vi "拉曼数据助手.vi"() -> ()   [LabVIEW 2020]
uses:
  <vilib>/Platform/TimedLoop/XDataNode/timing_clust.ctl
  <vilib>/Platform/TimedLoop/XDataNode/nitl_modes.ctl
  <vilib>/Platform/TimedLoop/XDataNode/wakeup.ctl
  <vilib>/picture/cartesn2.llb/XY Plot Type.ctl
  <vilib>/Instr/_visa.llb/VISA Configure Serial Port (Instr).vi
  <vilib>/Platform/TimedLoop/XDataNode/XDataNode.xnode
  <vilib>/Platform/TimedLoop/XDataNode/XDNodeRunTimeDep.lvlib
  <vilib>/Analysis/NI_AALPro.lvlib
  <vilib>/gmath/NI_Gmath.lvlib
panel:
  out "Window":bool
  out "配置文件路径":path
  out "偏移量":i32
  out "峰值范围":i32[][](array[numeric])
  out "λ picture":picture caption="新图片"
  out "pixel picture":picture
  in  "导出图像":bool
  in  "导出图像路路径":path caption="PNG图像文件路径"
  in  "自动寻峰":bool
  in  "关闭串口并退出":bool
  out "Debug状态":T1
  out "r^2":dbl caption="标定拟合 r" format="%.7g"
  in  "峰值波长":dbl[](array[numeric])=[0.0, 0.0]
  in  "峰值Pixel":dbl[](array[numeric])
  in  "自动转换":enum32{"Item 0", "Item 1"}(radio)
  out "波形XY图":T2
  in  "cartesian axis attributes":T3={"x minimum"=0.0, "x maximum"=0.0, "x log?"=FALSE, "x precision"=1, "x format"=enum."Decimal", "y minimum"=0.0, "y maximum"=0.0, "y log?"=FALSE, "y precision"=1, "y format"=enum."Decimal"} caption="直角坐标属性" {"x minimum" format="%0.2f"; "x maximum" format="%0.2f"; "y minimum" format="%0.2f"; "y maximum" format="%0.2f"}
  out "X轴":i32[](array[numeric])
  in  "导出文本":bool
  in  "数据存储路径":path=path "test.xlsx" caption="数据文件名"
  in  "暗背景扣除":bool
  in  "暗背景采集":bool
  out "暗背景":i64[](array[numeric])
  in  "确定":bool
  in  "时间单位":enum32{"Item 0", "Item 1"}(radio)
  in  "积分时间":dbl[unit]=0.1
  in  "Stop":bool
  out "采集状态":bool
  in  "波特率 (9600)":u32=9600 caption="波特率(9600)"
  in  "串口名":T4 caption="CCD检测器串口名"
  in  "开始":T5
  # "乙醇标定峰值 / pixel"
  # "2"
  # "-1"
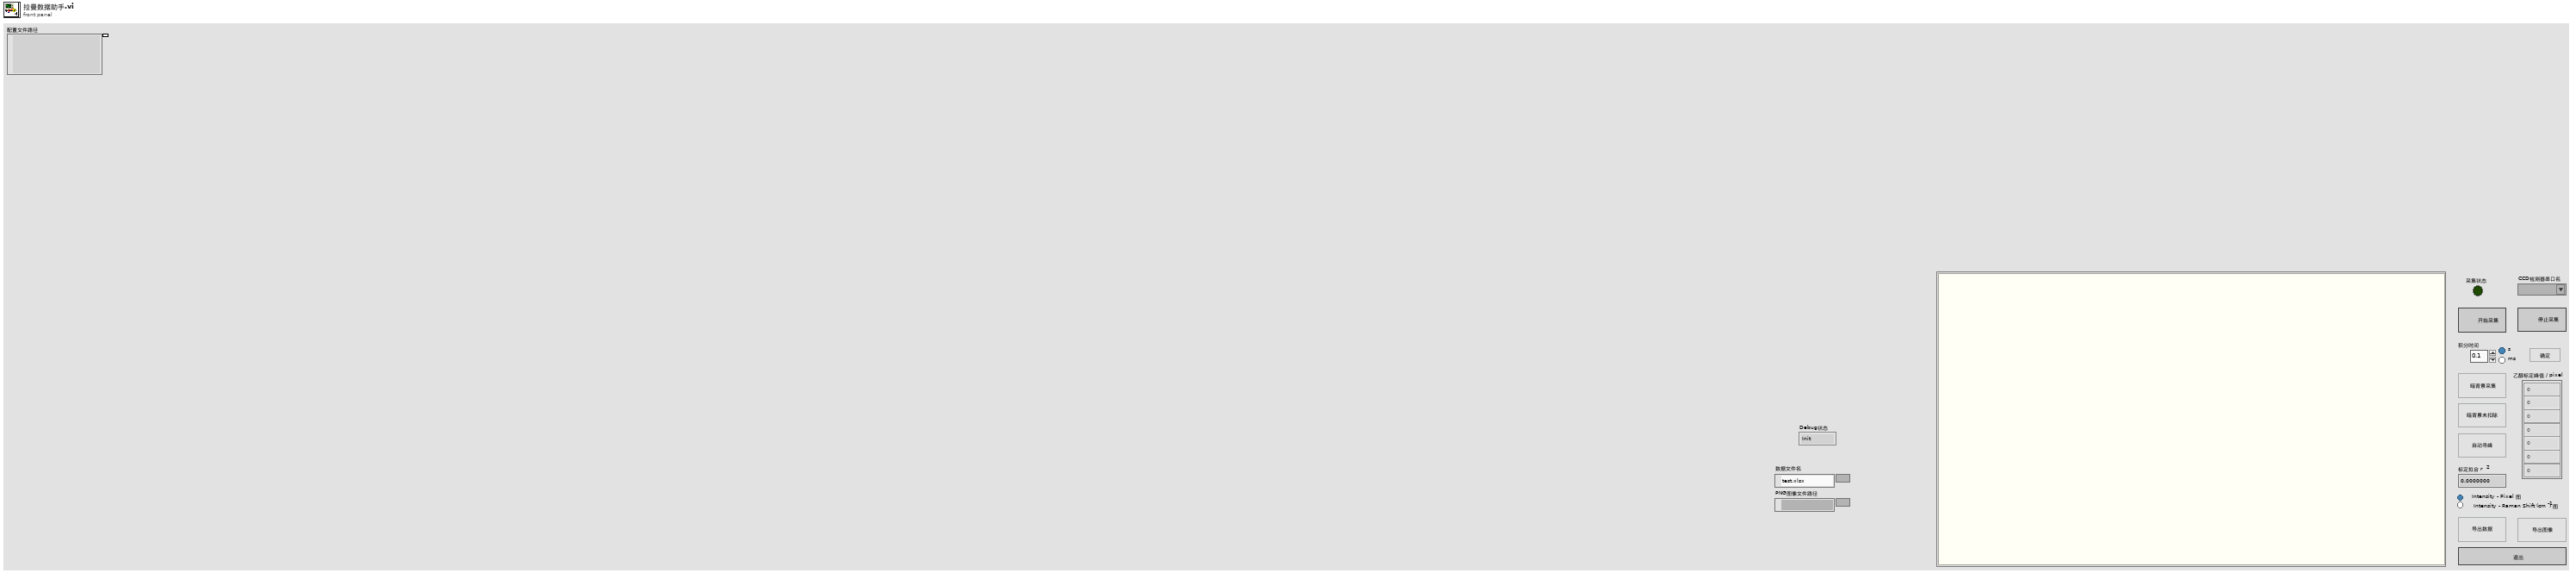
[diagram p1: front panel]
types:
  T1 = typedef "状态机.ctl" = enum16{"Init", "Wait", "GetData", "Exit"}
  T2 = typedef "？？.ctl" = picture
  T3 = cluster{"x minimum":dbl, "x maximum":dbl, "x log?":bool, "x precision":u8, "x format":enum8{"Decimal", "Scientific", "Engineering", "Binary", "Octal", "Hex"}, "y minimum":dbl, "y maximum":dbl, "y log?":bool, "y precision":u8, "y format":enum8{"Decimal", "Scientific", "Engineering", "Binary", "Octal", "Hex"}}
  T4 = typedef "控件 1.ctl" = refnum<visa-resource-name>
  T5 = typedef "1.ctl" = bool
  T6 = enum16{"open", "replace", "create", "open or create", "replace or create", "replace or create with confirmation"}
  T7 = cluster{"Font Name:":string, "Size":i16, "Strikeout?":bool, "Italic?":bool, "Underline?":bool, "Outline?":bool, "Shadow?":bool, "Bold?":bool}
  T8 = enum16{"User-specified Font", "Application Font", "System Font", "Dialog Font"}
  T9 = enum16{"None", "Stacked", "Clockwise", "Counterclockwise"}
  T10 = typedef "XY Plot Type.ctl" = enum16{"points", "squares", "circles", "connected points", "connected squares", "connected circles", "comb plot", "sized scatter plot", "sized-colored scatter plot", "min-max lines"}
  T11 = cluster{"plot color":u32, "XY plot type":T10, "baseline":dbl}
  T12 = cluster{"line color":u32, "text color":u32, "tick length(3)":i16, "crossing axes":bool, "visible grid?":bool}
  T13 = typedef "XDNodeRunTimeDep.lvlib/timing_clust.ctl" = cluster{"Expected End [f-1]":u64, "Actual End [f-1]":u64, "Finished Late? [f-1]":bool, "Expected End [i-1]":u64, "Actual End [i-1]":u64, "Finished Late? [i-1]":bool, "Expected Start [i]":u64, "Actual Start [i]":u64, "Expected Start [f]":u64, "Actual Start [f]":u64, "Source Name":string, "Structure Name":string, "Period":i64, "Deadline":i64, "Offset":i64, "Start":i64, "Priority":i32, "Timeout":i32, "Mode":T14, "Wakeup Reason":T15, "Error":errorcluster, "Source Type":string, "Secondary Source Type":string, "Global End Time":u64, "Global Start Time":u64, "Frame Duration":u64, "Iteration Duration":u64, "Assigned CPU":i32, "I/O Scan Engine Mode":u32}
  T14 = typedef "XDNodeRunTimeDep.lvlib/nitl_modes.ctl" = enum32{"No Change", "Process missed periods, maintain original phase", "Discard missed periods, maintain original phase", "Process missed periods, ignore original phase", "Discard missed periods, ignore original phase"}
  T15 = typedef "XDNodeRunTimeDep.lvlib/wakeup.ctl" = enum32{"Normal", "Aborted", "Asynchronous wakeup", "Timing source error", "Timed loop error", "Timeout"}
  T16 = cluster{i32, i32, i32, i32, i32, i32, i32, i32, i32, i32, i32, i32, i32, i32}
  T17 = typedef "imagedata.ctl" = cluster{"image type":i32, "image depth":i32, "image":u8[], "mask":u8[], "colors":u32[], "Rectangle":cluster{"left":i16, "top":i16, "right":i16, "bottom":i16}}
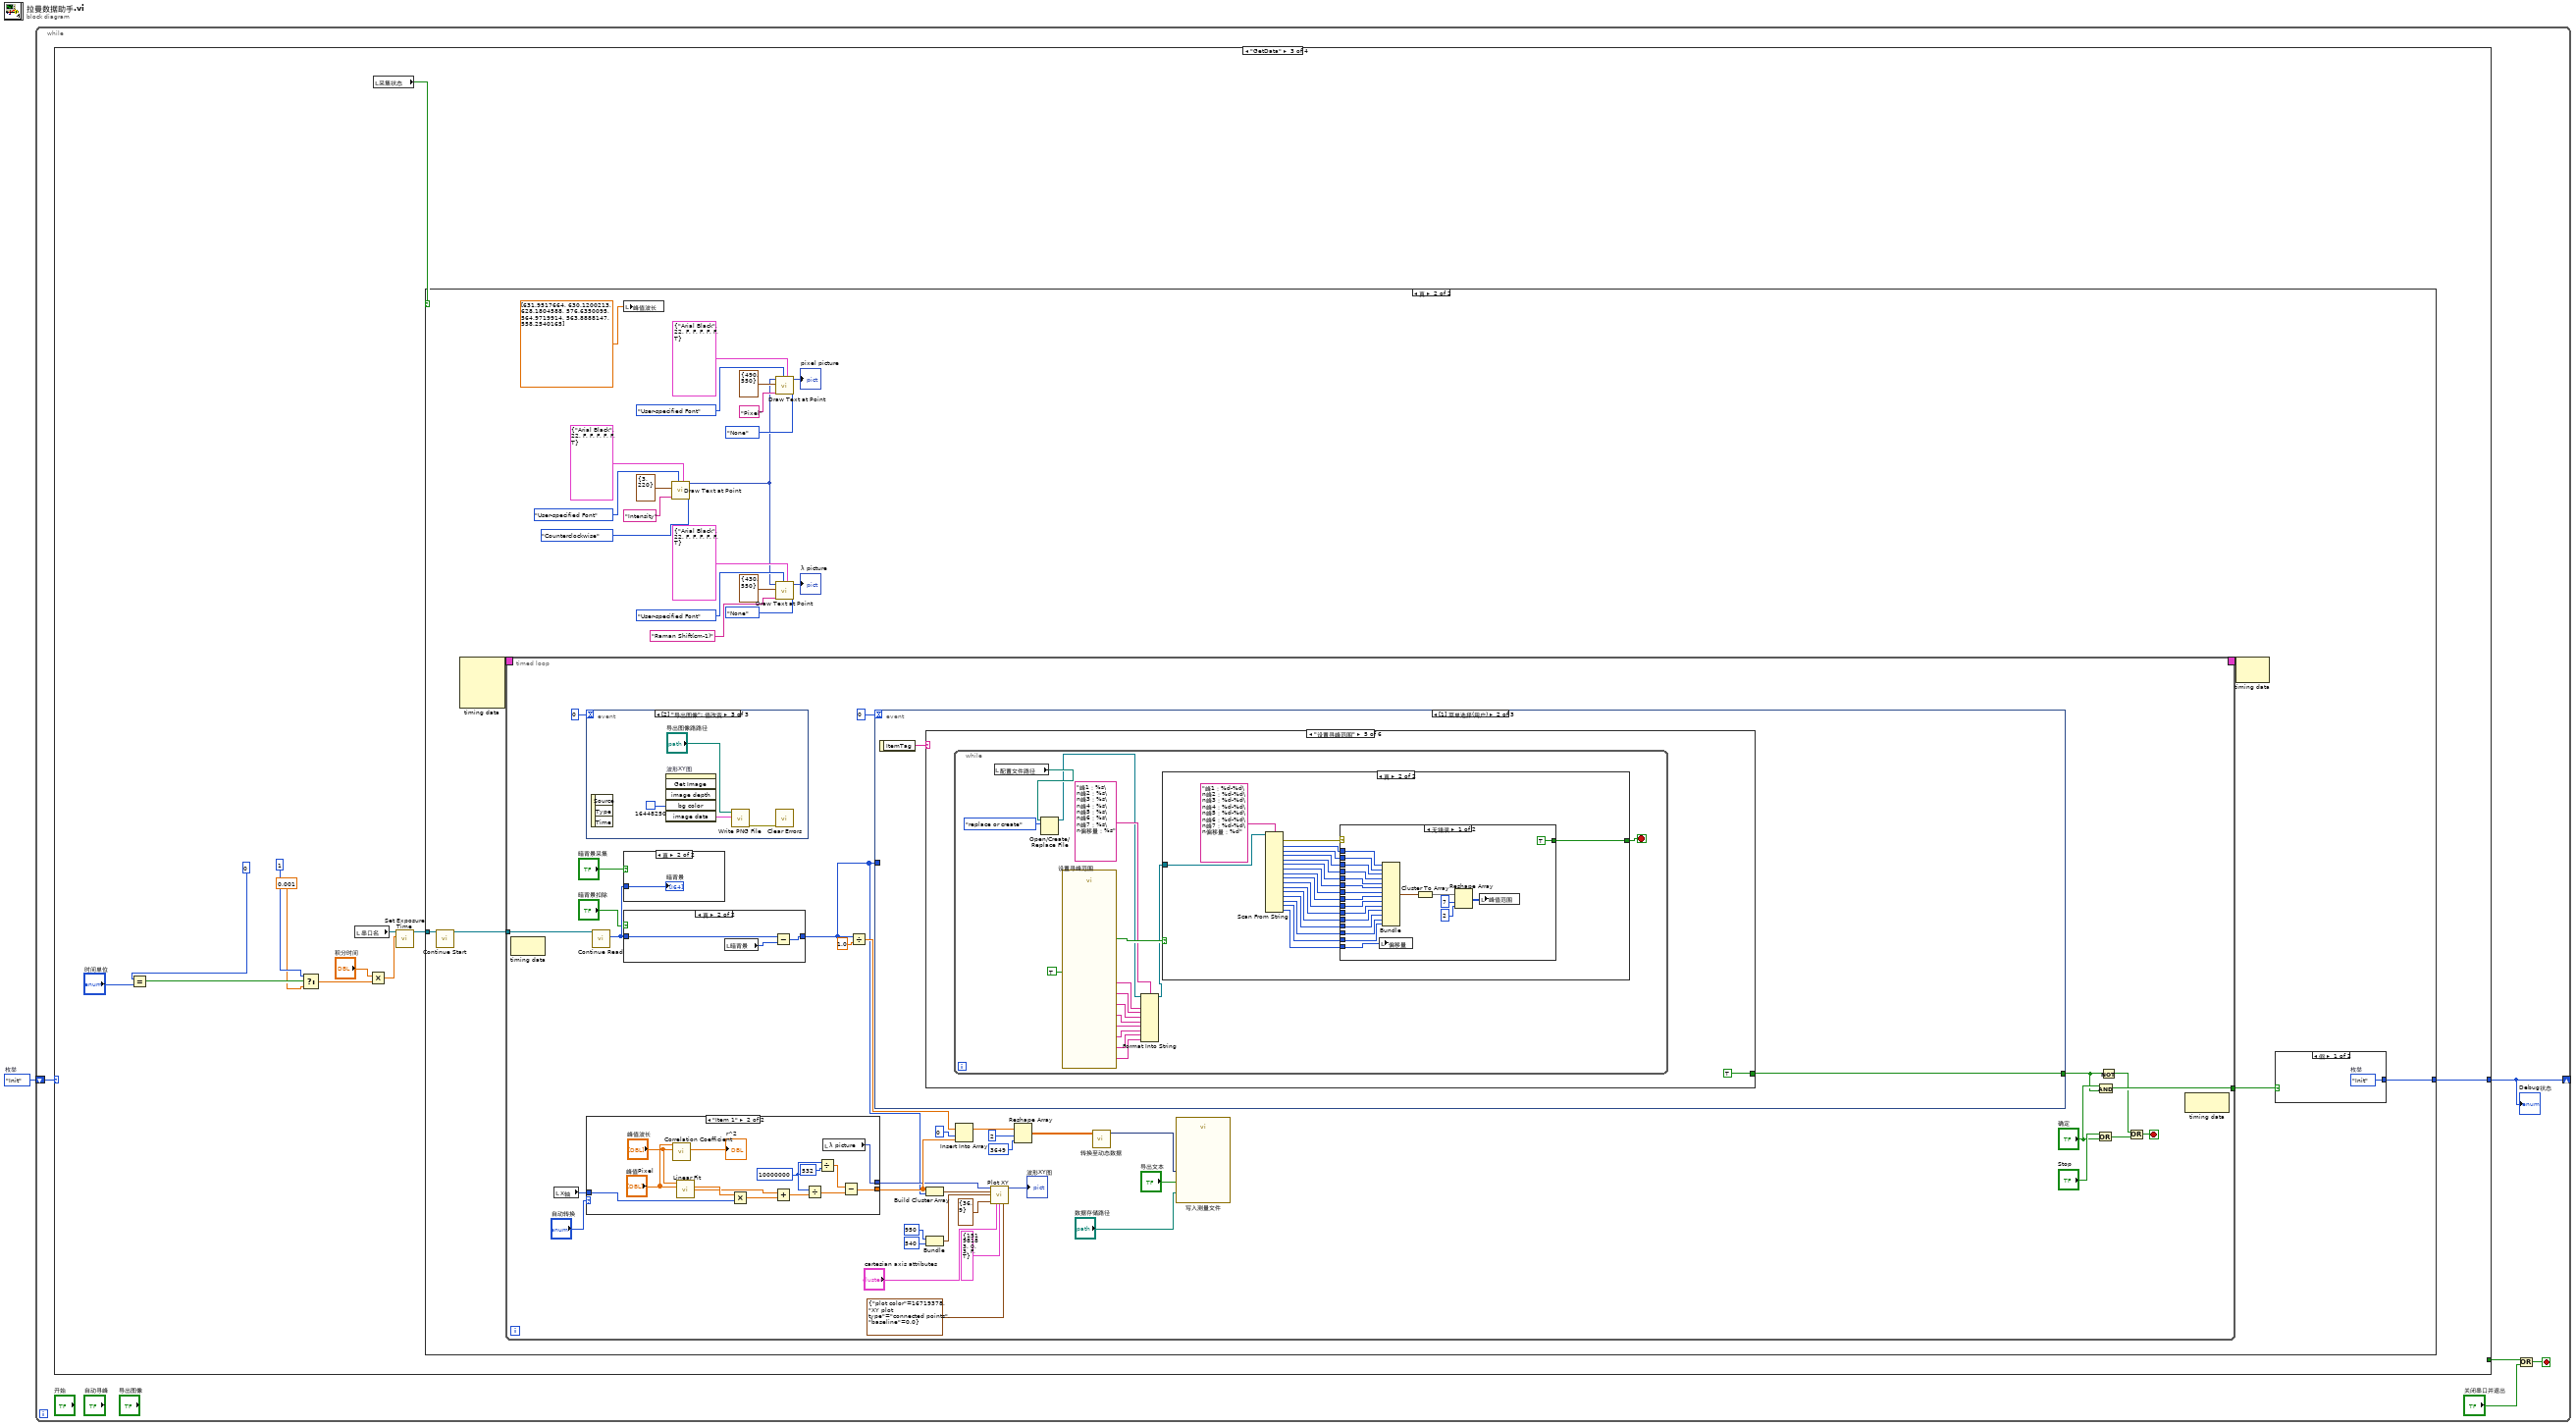
[diagram p0: block diagram]
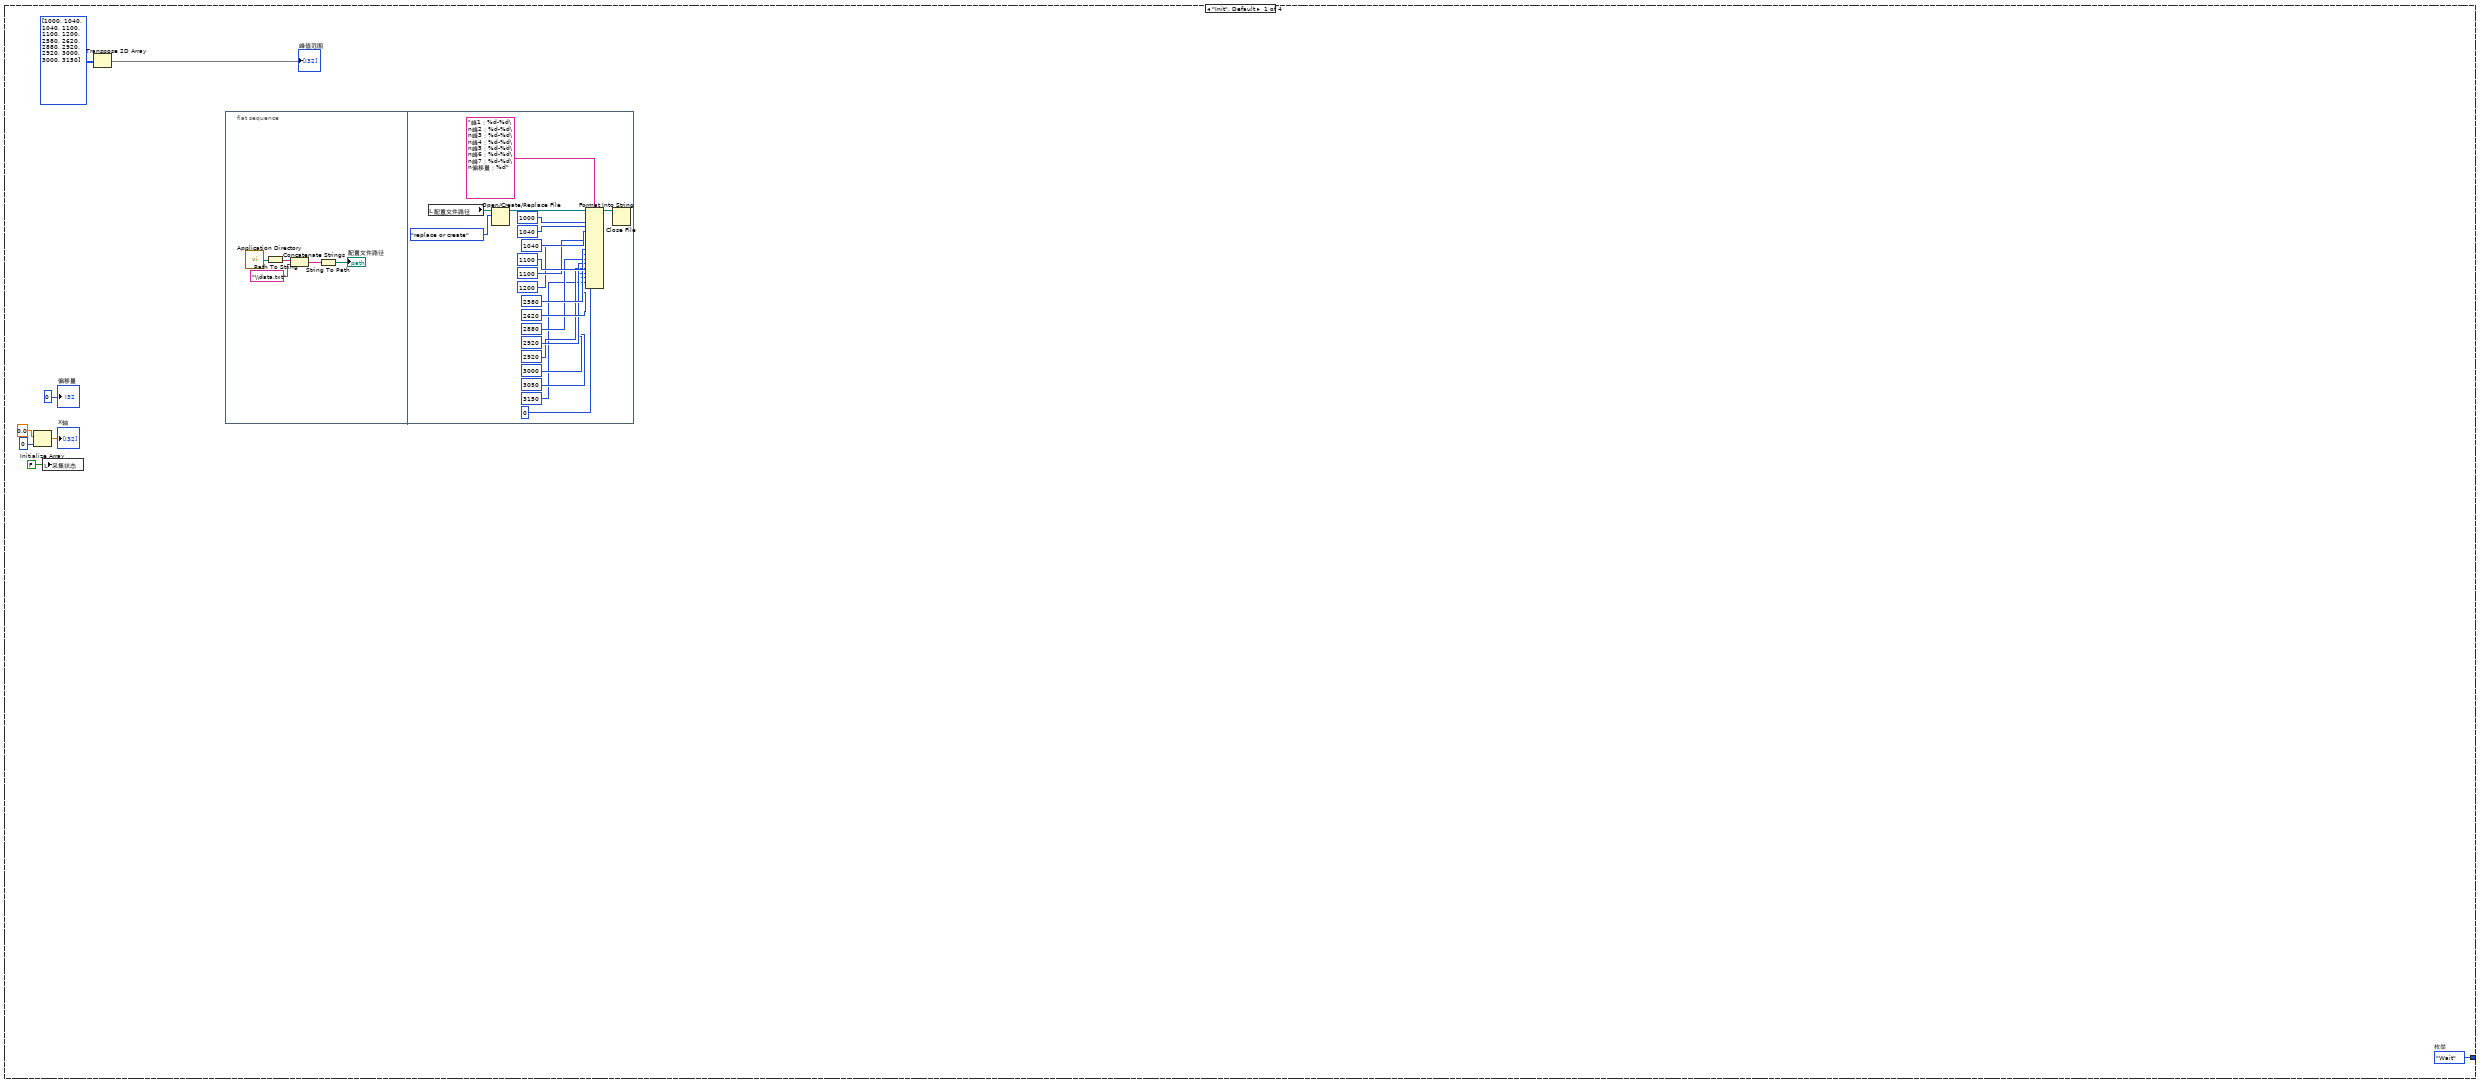
[diagram p2: hidden frame]
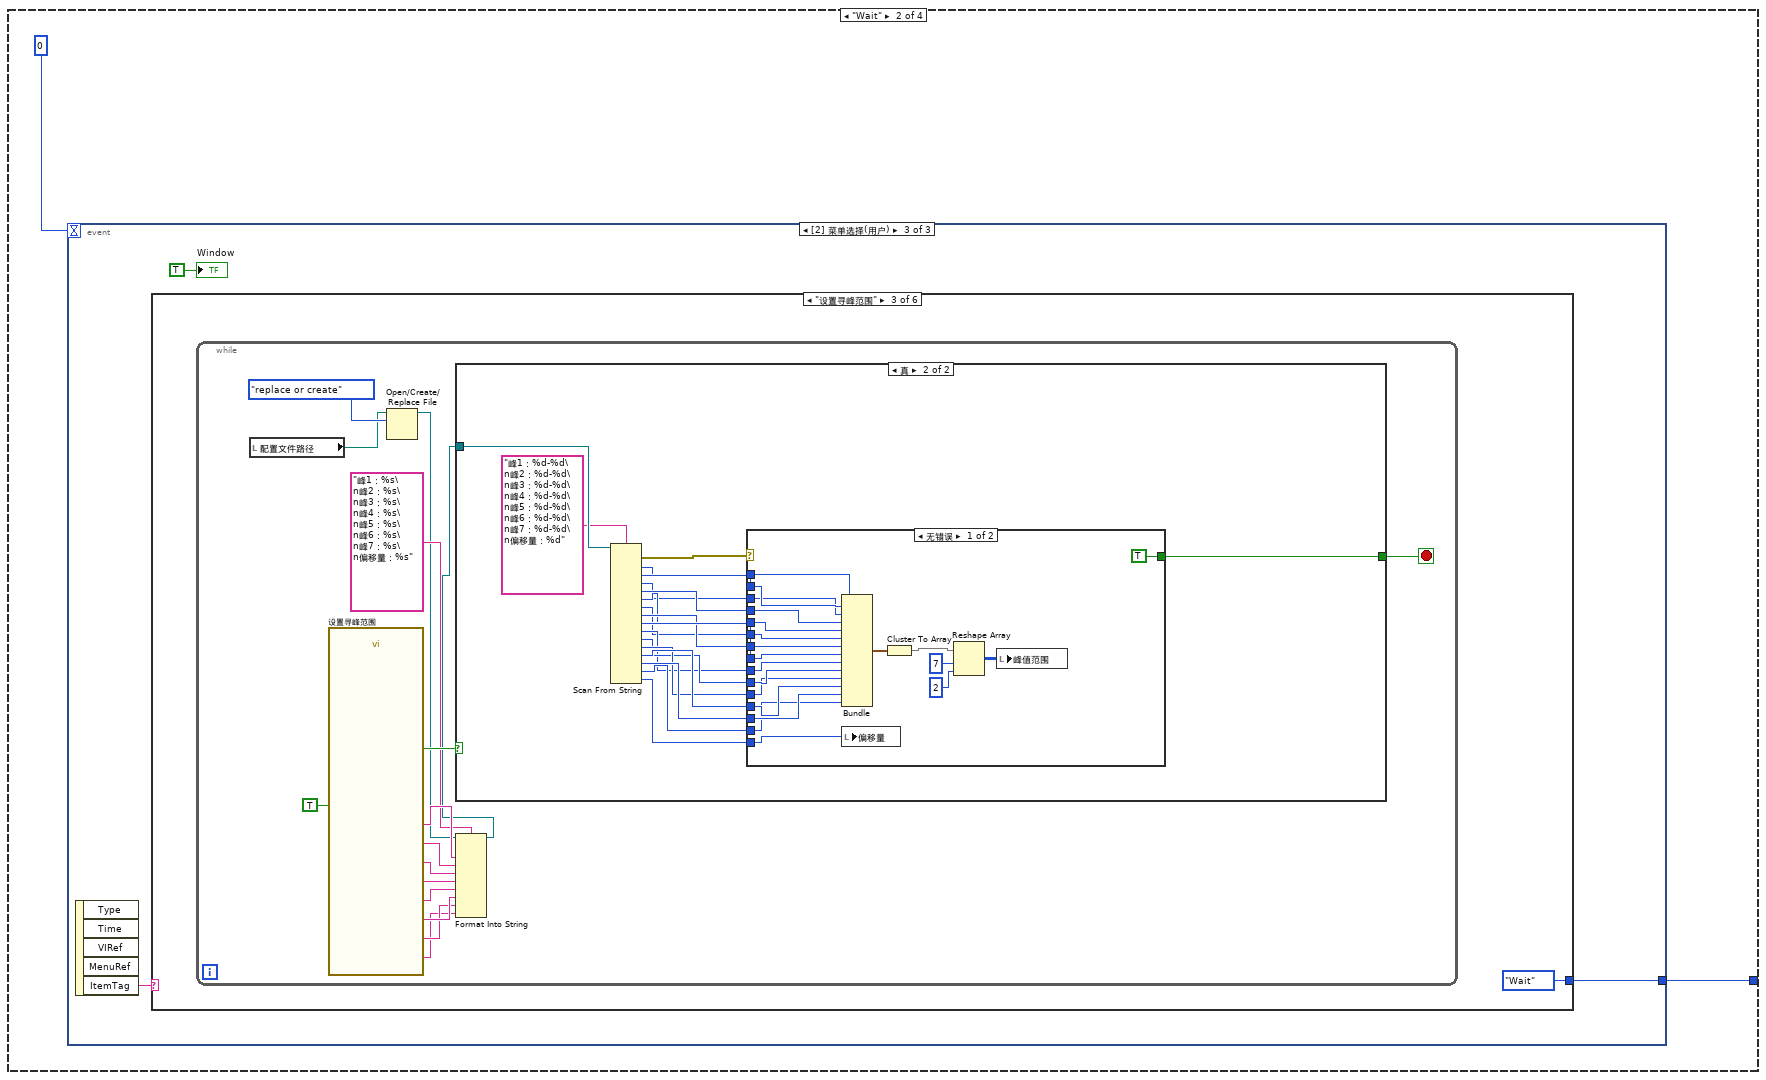
[diagram p3: hidden frame]
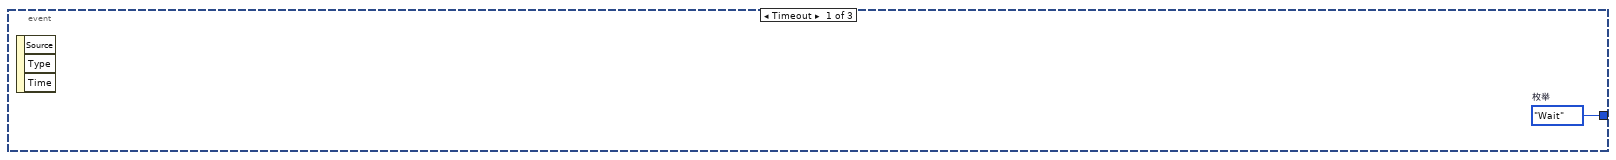
[diagram p4: hidden frame]
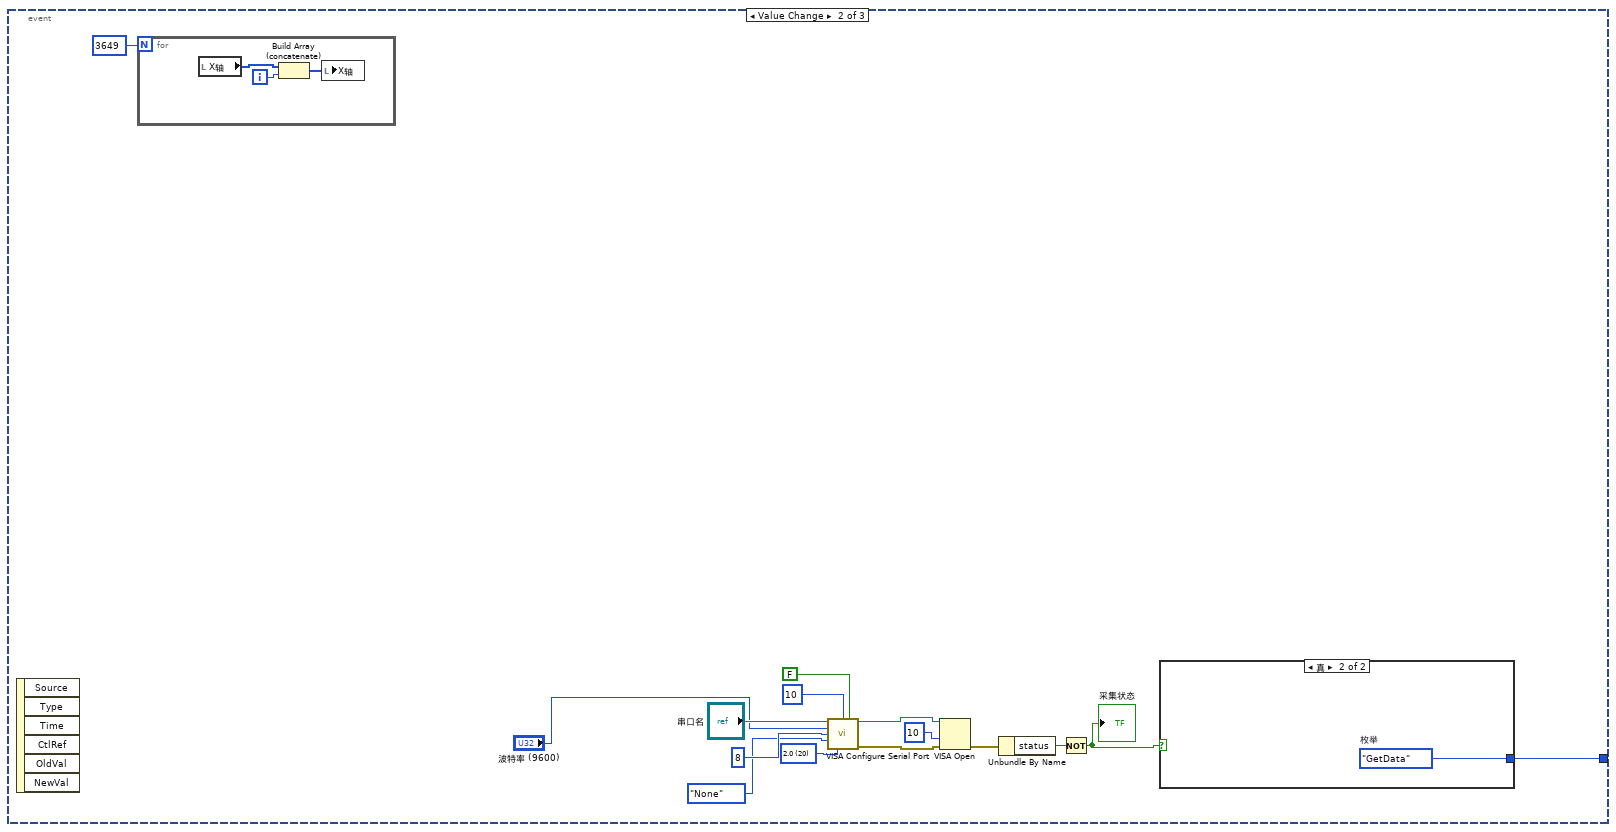
[diagram p5: hidden frame]
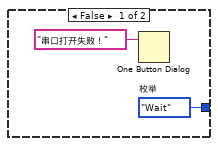
[diagram p6: hidden frame]
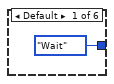
[diagram p7: hidden frame]
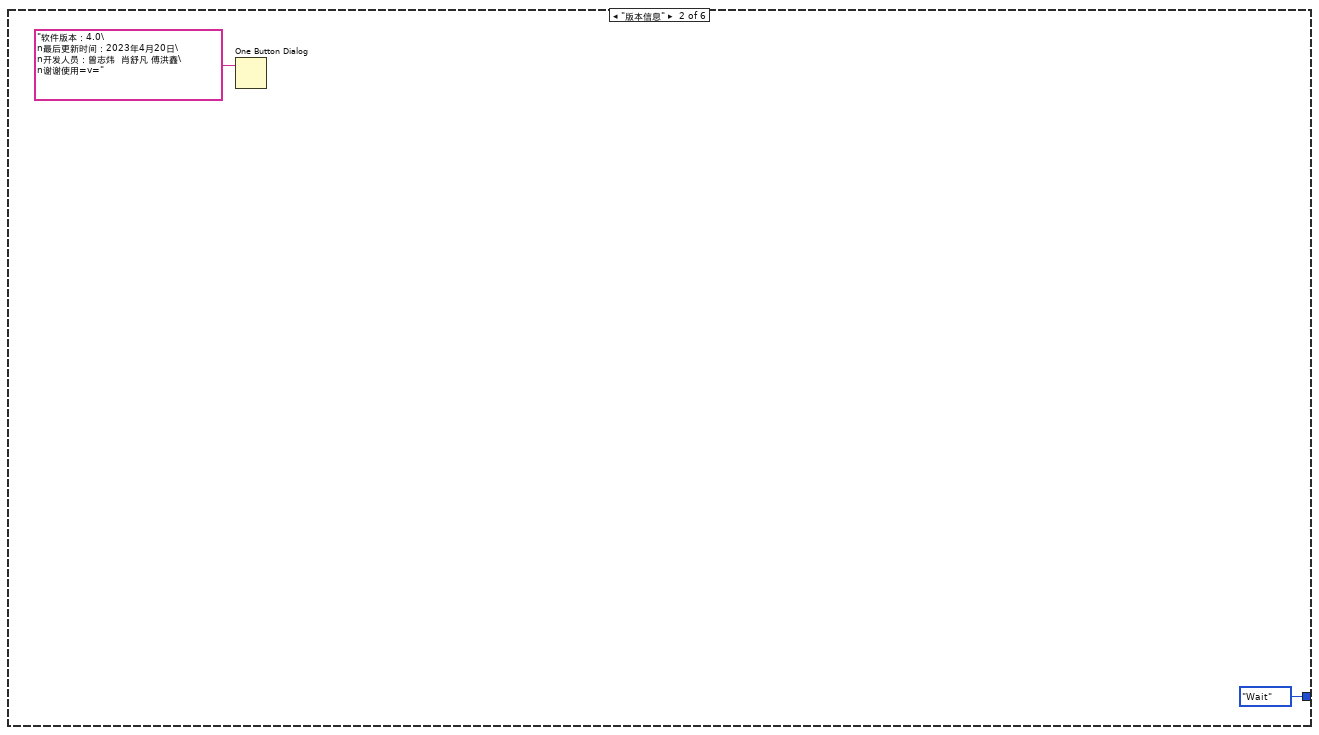
[diagram p8: hidden frame]
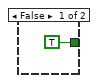
[diagram p9: hidden frame]
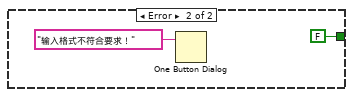
[diagram p10: hidden frame]
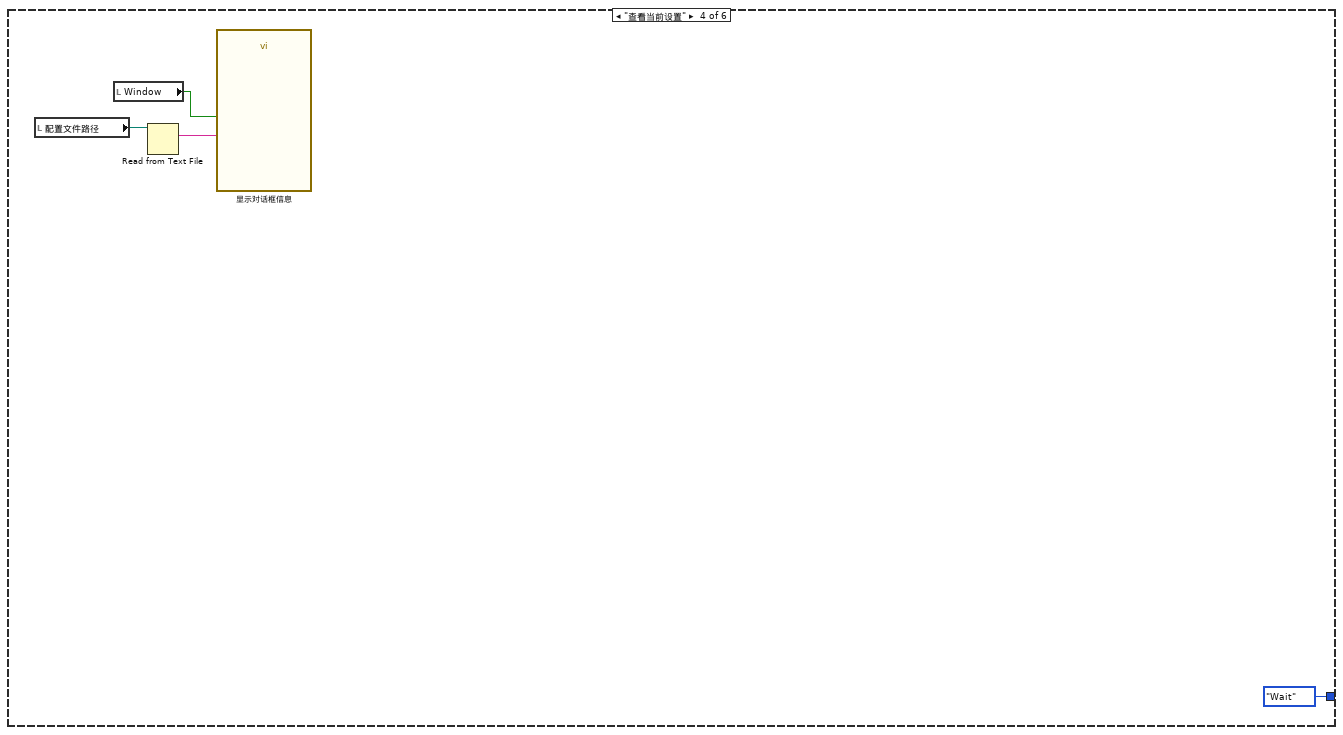
[diagram p11: hidden frame]
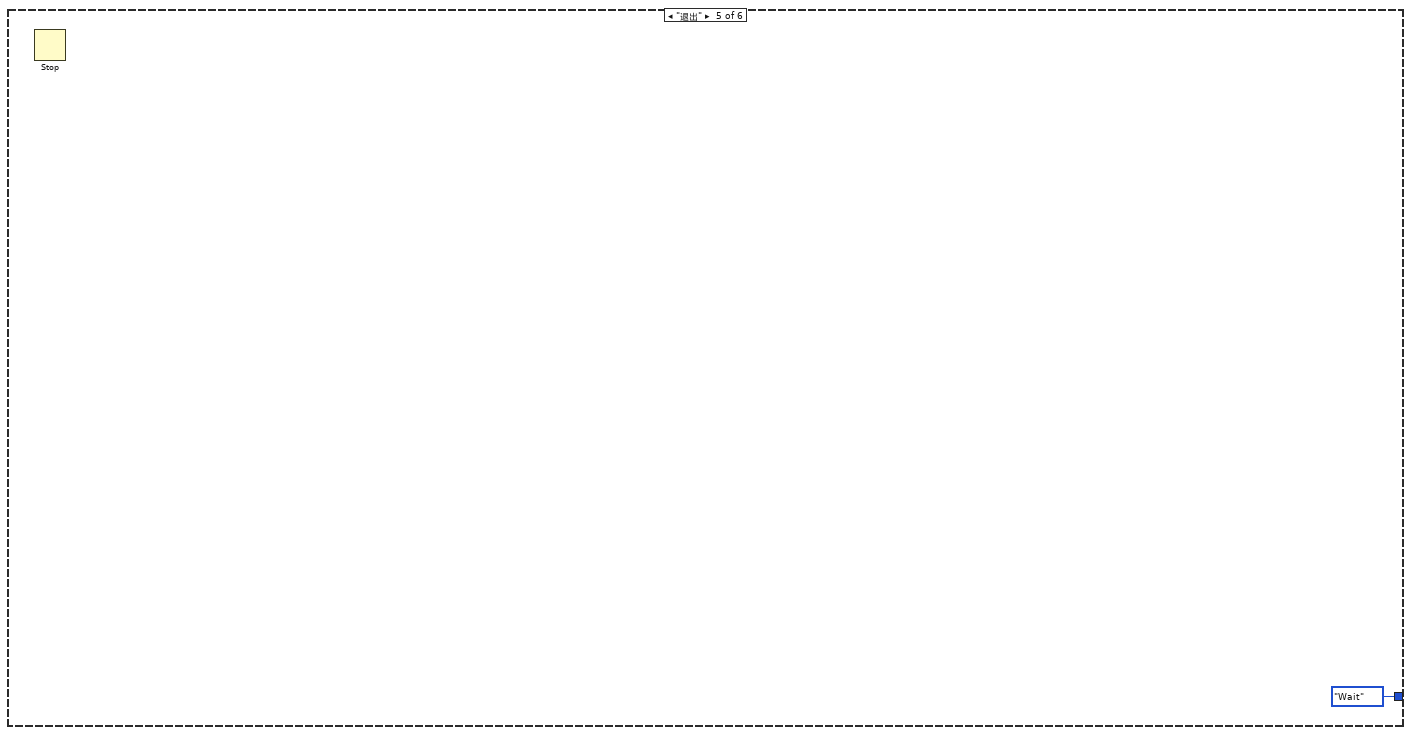
[diagram p12: hidden frame]
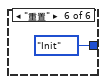
[diagram p13: hidden frame]
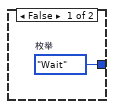
[diagram p14: hidden frame]
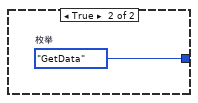
[diagram p15: hidden frame]
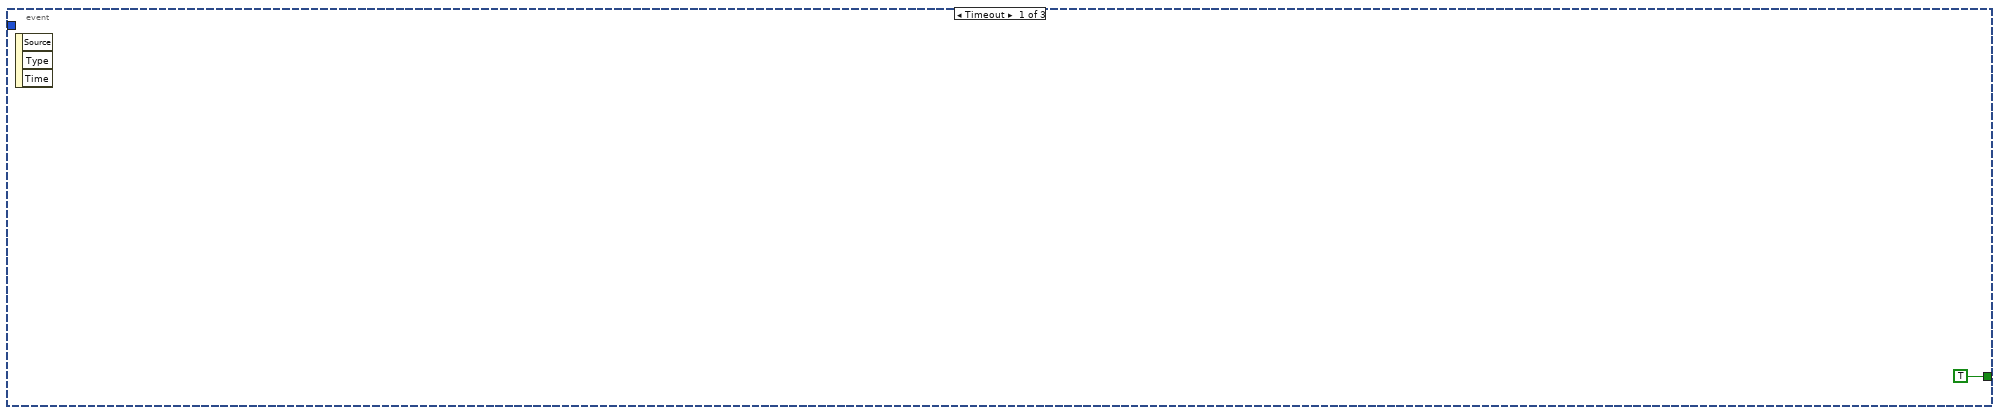
[diagram p16: hidden frame]
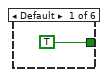
[diagram p17: hidden frame]
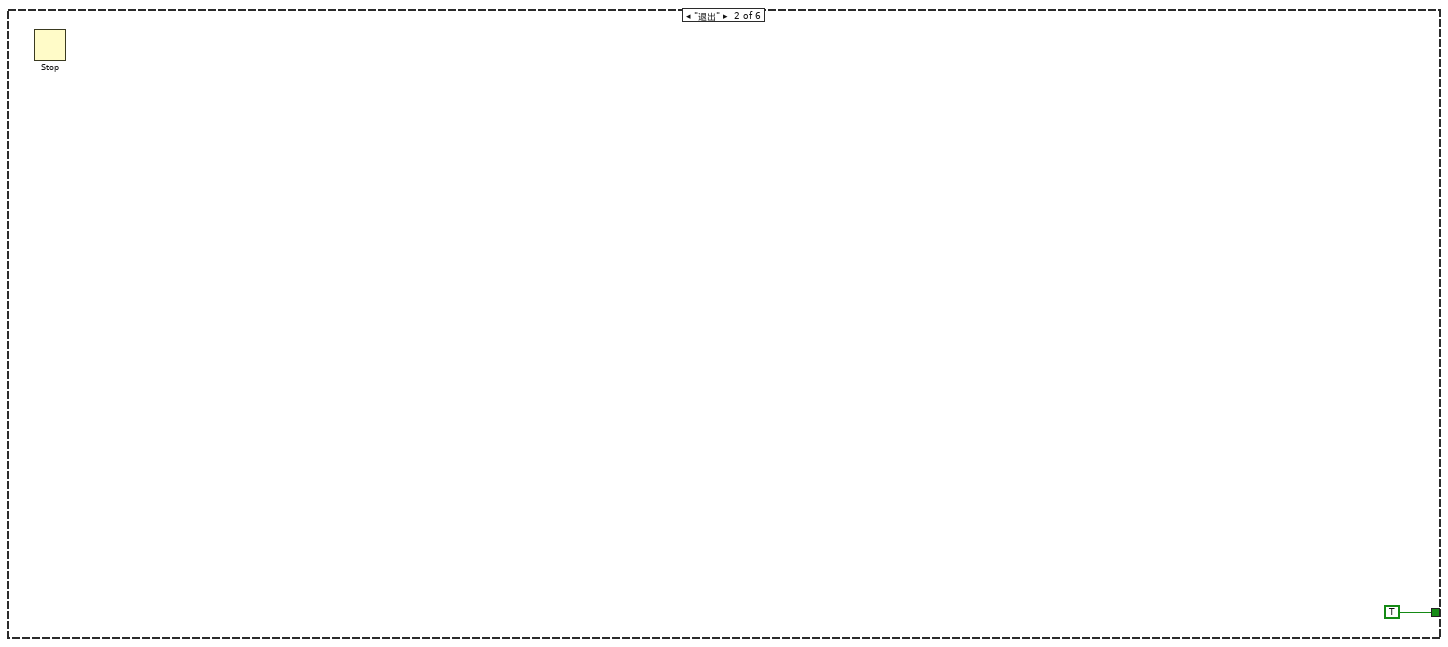
[diagram p18: hidden frame]
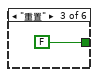
[diagram p19: hidden frame]
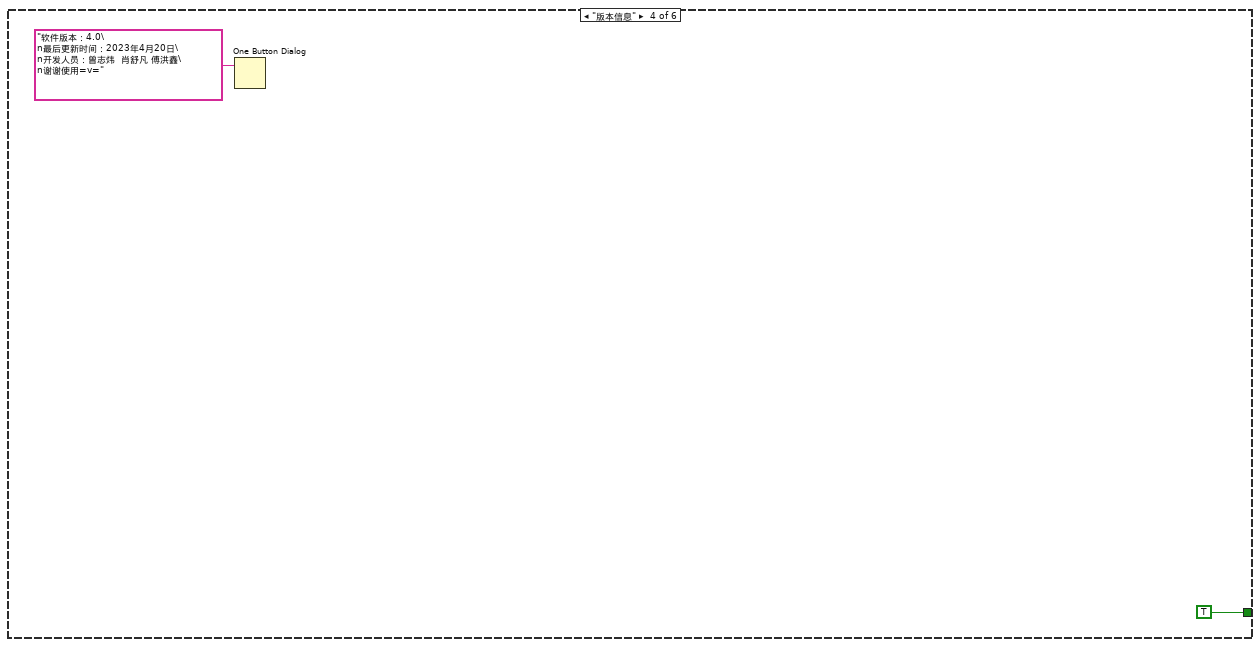
[diagram p20: hidden frame]
diagram:
  w1 = 状态机."Init"  # 枚举
  n1 = while {
    shift-right: [w5] -> _
    shift-left: w1 -> [w6]
    stop <- w2 stop-if-true
    n2 = case shown="\"GetData\"" w6 {
      tunnel: [w13 w40 w145 w422] -> w5
      tunnel: [_ _ _ FALSE] -> w4
      frame "Init", Default {
        w13 = 状态机."Wait"  # 枚举
        n3 = Initialize Array(0.0 ("元素"), 0 ("维数大小")) -> (→"X轴":dbl[])
        n4 = local write "采集状态"(FALSE ("打开状态")) -> ()
        n5 = Transpose 2D Array(2D array=i32[][] [[1000, 1040], [1040, 1100], [1100, 1200], [2580, 2620], [2880, 2920], [2920, 3000], [3000, 3150]]) -> (transposed array=→"峰值范围":i32[][])
        n6 = flat-sequence {
          frame #0 {
            n7 = call <vilib>:"Application Directory.vi"() -> ("Application Directory"=w19:path)
            n8 = Path To String(path=w19) -> (string=w18:string)
            n9 = Concatenate Strings(w18, "\\data.txt" ("字符串")) -> (w16:string)
            n10 = String To Path(string=w16) -> (path=→"配置文件路径":path)
          }
          frame #1 {
            n11 = local read "配置文件路径"() -> (w37:path)
            n12 = Open/Create/Replace File(file path (use dialog)=w37, operation (0:open)=T6."replace or create" ("操作(0:open)")) -> (refnum out=w38:refnum<file>)  [unwired: 4 in, 2 out]
            n13 = Format Into String(format string="峰1：%d-%d\n峰2：%d-%d\n峰3：%d-%d\n峰4：%d-%d\n峰5：%d-%d\n峰6：%d-%d\n峰7：%d-%d\n偏移量：%d" ("格式字符串"), initial string=w38, 1000 ("输入 1"), 1040 ("输入 2"), 1040, 1100 ("输入 4"), 1100 ("输入 5"), 1200 ("输入 6"), 2580 ("输入 7"), 2620 ("输入 8"), 2880 ("输入 9"), 2920 ("输入 10"), 2920 ("输入 11"), 3000 ("输入 12"), 3050 ("输入 13"), 3150 ("输入 14"), 0 ("输入 15")) -> (resulting string=w39:refnum<file>)  [unwired: 1 in, 1 out]
            n14 = Close File(refnum=w39) -> ()  [unwired: 1 in, 2 out]
          }
        }
        "偏移量" <- 0
      }
      frame "Wait" {
        n15 = event shown="[2] 菜单选择(用户)" {
          selector: _ -> [_ _ _]
          dyn-events: _ -> [_ _ _]
          timeout: 0 -> [_ _ _]
          tunnel: [w42 w57 w64] -> w40
          event Timeout {
            w42 = 状态机."Wait"  # 枚举
            n16 = event-data() -> ()  [unwired: 1 in, 3 out]
          }
          event Value Change {
            w44 = u16 20 items=["1.0"=10, "1.5"=15, "2.0"=20] ("stop bits (10: 1 bit)")
            n17 = event-data() -> ()  [unwired: 1 in, 6 out]
            n18 = for {
              N: 3649 -> [_]
              i -> [w59]
              n19 = local read "X轴"() -> (w60:i32[])
              n20 = Build Array (concatenate)(w60, w59) -> (w58:i32[])
              n21 = local write "X轴"(w58) -> ()
            }
            n22 = call-poly "VISA Configure Serial Port"("VISA resource name"="串口名", "termination char\n(0xA = '\\n' = LF)"=u8 10 ("termination char\n(0xA = '\\n' = LF)"), "Enable Termination\nChar (T)"=FALSE ("Enable Termination\nChar (T)"), "baud rate (9600)"="波特率 (9600)", "data bits (8)"=u16 8, "parity (0:none)"=enum16{"None", "Odd", "Even", "Mark", "Space"}."None", "stop bits (10: 1 bit)"=w44) -> ("VISA resource name out"=w52:refnum<visa-resource-name>, "error out"=w51:errorcluster)  [unwired: 7 in]
            n23 = VISA Open(access mode=10, error in (no error)=w51, VISA resource name=w52) -> (error out=w50:errorcluster)  [unwired: 2 in, 1 out]
            n24 = Unbundle By Name(w50) -> ("status"=w55:bool)
            n25 = Not(x=w55) -> (.not. x?=w54:bool)
            "采集状态" <- w54
            n26 = case shown="真" w54 {
              tunnel: [w61 w63] -> w57
              frame False {
                w61 = 状态机."Wait"  # 枚举
                n27 = One Button Dialog(message="串口打开失败！" ("消息")) -> ()  [unwired: 1 in, 1 out]
              }
              frame True {
                w63 = 状态机."GetData"  # 枚举
              }
            }
          }
          event Menu Selection (User) {
            n28 = event-data() -> ("ItemTag"=w66:string)  [unwired: 1 in, 4 out]
            n29 = case shown="\"设置寻峰范围\"" w66 {
              tunnel: [状态机."Wait" ("枚举") 状态机."Wait" ("枚举") 状态机."Wait" ("枚举") 状态机."Wait" ("枚举") 状态机."Wait" ("枚举") 状态机."Init" ("枚举")] -> w64
              frame Default {
              }
              frame "版本信息" {
                n30 = One Button Dialog(message="软件版本：4.0\n最后更新时间：2023年4月20日\n开发人员：曾志炜  肖舒凡 傅洪鑫\n谢谢使用=v=" ("消息")) -> ()  [unwired: 1 in, 1 out]
              }
              frame "设置寻峰范围" {
                n31 = while {
                  stop <- w75 stop-if-true
                  n32 = local read "配置文件路径"() -> (w73:path)
                  n33 = call "设置寻峰范围"("Enable"=TRUE) -> ("偏移量"=w77:string, "峰7"=w78:string, "峰6"=w79:string, "峰5"=w80:string, "峰4"=w81:string, "峰3"=w82:string, "峰2"=w83:string, "峰1"=w84:string, "确定"=w86:bool)  [unwired: 9 in, 1 out]
                  n34 = Open/Create/Replace File(file path (use dialog)=w73, operation (0:open)=T6."replace or create" ("操作(0:open)")) -> (refnum out=w72:refnum<file>)  [unwired: 4 in, 2 out]
                  n35 = Format Into String(format string="峰1：%s\n峰2：%s\n峰3：%s\n峰4：%s\n峰5：%s\n峰6：%s\n峰7：%s\n偏移量：%s" ("格式字符串"), initial string=w72, w84, w83, w82, w81, w80, w79, w78, w77) -> (resulting string=w71:refnum<file>)  [unwired: 1 in, 1 out]
                  n36 = case shown="真" w86 {
                    tunnel: w71 -> [_ w106]
                    tunnel: [TRUE w88] -> w75
                    frame False {
                    }
                    frame True {
                      n37 = Scan From String("峰1：%d-%d\n峰2：%d-%d\n峰3：%d-%d\n峰4：%d-%d\n峰5：%d-%d\n峰6：%d-%d\n峰7：%d-%d\n偏移量：%d" ("格式字符串"), w106) -> (w105:errorcluster, output 1=w91:i32, output 2=w92:i32, output 3=w93:i32, output 4=w94:i32, output 5=w95:i32, output 6=w96:i32, output 7=w97:i32, output 8=w98:i32, output 9=w99:i32, output 10=w100:i32, output 11=w101:i32, output 12=w102:i32, output 13=w103:i32, output 14=w104:i32, output 15=w90:i32)  [unwired: 16 in, 1 out]
                      n38 = case shown="无错误" w105 {
                        tunnel: w90 -> [w127 _]
                        tunnel: w91 -> [w126 _]
                        tunnel: w92 -> [w125 _]
                        tunnel: w93 -> [w124 _]
                        tunnel: w94 -> [w123 _]
                        tunnel: w95 -> [w122 _]
                        tunnel: w96 -> [w121 _]
                        tunnel: w97 -> [w120 _]
                        tunnel: w98 -> [w119 _]
                        tunnel: w99 -> [w118 _]
                        tunnel: w100 -> [w117 _]
                        tunnel: w101 -> [w116 _]
                        tunnel: w102 -> [w115 _]
                        tunnel: w103 -> [w114 _]
                        tunnel: w104 -> [w113 _]
                        tunnel: [TRUE FALSE] -> w88
                        frame No Error {
                          n39 = Bundle(w126, w125, w124, w123, w122, w121, w120, w119, w118, w117, w116, w115, w114, w113) -> (w112:T16)  [unwired: 1 in]
                          n40 = local write "偏移量"(w127) -> ()
                          n41 = Cluster To Array(cluster=w112) -> (array=w111:i32[])
                          n42 = Reshape Array(w111, 7 ("维数大小"), 2 ("维数大小")) -> (w108:i32[][])
                          n43 = local write "峰值范围"(w108) -> ()
                        }
                        frame Error {
                          n44 = One Button Dialog(message="输入格式不符合要求！" ("消息")) -> ()  [unwired: 1 in, 1 out]
                        }
                      }
                    }
                  }
                }
              }
              frame "查看当前设置" {
                n45 = local read "配置文件路径"() -> (w133:path)
                n46 = local read "Window"() -> (w131:bool)
                n47 = Read from Text File(file (use dialog)=w133) -> (text=w132:string)  [unwired: 3 in, 3 out]
                n48 = call "显示对话框信息"("Enable"=w131, "Message"=w132) -> ()  [unwired: 8 in, 2 out]
              }
              frame "退出" {
                n49 = Stop() -> ()  [unwired: 1 in]
              }
              frame "重置" {
              }
            }
            "Window" <- TRUE
          }
        }
      }
      frame "GetData" {
        n50 = Equal?(x=0, y="时间单位") -> (x = y?=w141:bool)
        n51 = Select(t=1, s=w141, f=0.001) -> (s? t:f=w138:dbl)
        n52 = local read "串口名"() -> (w147:T4)
        n53 = Multiply(x="积分时间", y=w138) -> (x*y=w139:dbl[unit])
        n54 = local read "采集状态"() -> (w144:bool)
        n55 = call "Set Exposure Time.vi"("Exposure Time"=w139, "Com in"=w147) -> ("Com out"=w146:refnum<visa-resource-name>)  [unwired: 8 in, 1 out]
        n56 = case shown="真" w144 {
          tunnel: w146 -> [_ w173]
          tunnel: [w148 w171] -> w145
          frame False {
            w148 = 状态机."Wait"  # 枚举
          }
          frame True {
            n57 = call "Continue Start.vi"("Com in"=w173) -> ("Com out"=w172:refnum<visa-resource-name>)  [unwired: 9 in, 1 out]
            n58 = node-c288() -> (w170:T13)  [unwired: 4 in]
            n59 = timed-loop {
              tunnel: w172 -> [w212]
              timing: w170 -> [_]
              timing-out: [_] -> w169
              tunnel: [w180] -> w168
              stop <- w176 stop-if-true
              n60 = node-c288() -> ()  [unwired: 1 in, 1 out]
              n61 = local read "X轴"() -> (w190:i32[])
              n62 = event shown="[2] \"导出图像\": 值改变" {
                selector: _ -> [_ _ _]
                dyn-events: _ -> [_ _ _]
                timeout: 0 -> [_ _ _]
                event Timeout {
                  n63 = event-data() -> ()  [unwired: 1 in, 3 out]
                }
                event "Stop": Value Change {
                  n64 = event-data() -> ()  [unwired: 1 in, 3 out]
                  n65 = local write "采集状态"(FALSE ("采集状态")) -> ()
                }
                event "导出图像": Value Change {
                  n66 = event-data() -> ()  [unwired: 1 in, 3 out]
                  n67 = invoke on="波形XY图" class="Pict (严格)" method="Get Image"("bg color"=u32 16448250 ("背景色")) -> ("image data"=w392:T17)  [unwired: 5 in, 5 out]
                  n68 = call <vilib>:"Write PNG File.vi"("image data"=w392, "path to PNG file"="导出图像路路径") -> ("error out"=w391:errorcluster)  [unwired: 8 in, 1 out]
                  n69 = call <vilib>:"Clear Errors.vi"("error in (no error)"=w391) -> ()  [unwired: 5 in, 2 out]
                }
              }
              n70 = case shown="\"Item 1\"" "自动转换" {
                tunnel: w190 -> [w396 w410]
                tunnel: [w396 w404] -> w189
                tunnel: [w395 w397] -> w184
                frame "Item 0", Default {
                  n71 = local read "pixel picture"() -> (w395:picture)
                }
                frame "Item 1" {
                  w406 = 10000000
                  n72 = call <vilib>:"Correlation Coefficient.vi"("Y"="峰值波长", "X"="峰值Pixel") -> ("r^2"=→"r^2":dbl)  [unwired: 8 in, 1 out]
                  n73 = call <vilib>:"Linear Fit.vi"("Y"="峰值波长", "X"="峰值Pixel") -> ("slope"=w402:dbl, "intercept"=w401:dbl)  [unwired: 9 in, 3 out]
                  n74 = Multiply(x=w402, y=w410) -> (x*y=w409:dbl[])
                  n75 = Add(x=w401, y=w409) -> (x+y=w403:dbl[])
                  n76 = Divide(x=w406, y=w403) -> (x/y=w405:dbl[])
                  n77 = Divide(x=w406, y=532) -> (x/y=w407:dbl)
                  n78 = local read "λ picture"() -> (w397:picture)
                  n79 = Subtract(x=w407, y=w405) -> (x-y=w404:dbl[])
                }
              }
              n80 = call "Continue Read.vi"("Com in"=w212) -> ("Data"=w209:i64[])  [unwired: 8 in, 2 out]
              n81 = case shown="真" "暗背景采集" {
                tunnel: w209 -> [_ w415]
                frame False {
                }
                frame True {
                  "暗背景" <- w415
                }
              }
              n82 = case shown="真" "暗背景扣除" {
                tunnel: w209 -> [w411 w414]
                tunnel: [w411 w413] -> w182
                frame False {
                }
                frame True {
                  n83 = local read "暗背景"() -> (w412:i64[])
                  n84 = Subtract(x=w414, y=w412) -> (x-y=w413:i64[])
                }
              }
              n85 = Divide(x=w182, y=1.0) -> (x/y=w187:dbl[])
              n86 = event shown="[1] 菜单选择(用户)" {
                selector: _ -> [_ _ _]
                dyn-events: _ -> [_ _ _]
                timeout: 0 -> [_ _ _]
                tunnel: w182 -> [_ _ w286]
                tunnel: [TRUE w214 TRUE] -> w179
                event Timeout {
                  n87 = event-data() -> ()  [unwired: 1 in, 3 out]
                }
                event Menu Selection (User) {
                  n88 = event-data() -> ("ItemTag"=w215:string)  [unwired: 1 in]
                  n89 = case shown="\"设置寻峰范围\"" w215 {
                    tunnel: [TRUE TRUE FALSE TRUE TRUE TRUE] -> w214
                    frame Default {
                    }
                    frame "退出" {
                      n90 = Stop() -> ()  [unwired: 1 in]
                    }
                    frame "重置" {
                    }
                    frame "版本信息" {
                      n91 = One Button Dialog(message="软件版本：4.0\n最后更新时间：2023年4月20日\n开发人员：曾志炜  肖舒凡 傅洪鑫\n谢谢使用=v=" ("消息")) -> ()  [unwired: 1 in, 1 out]
                    }
                    frame "设置寻峰范围" {
                      n92 = while {
                        stop <- w226 stop-if-true
                        n93 = local read "配置文件路径"() -> (w224:path)
                        n94 = Open/Create/Replace File(file path (use dialog)=w224, operation (0:open)=T6."replace or create" ("操作(0:open)")) -> (refnum out=w223:refnum<file>)  [unwired: 4 in, 2 out]
                        n95 = call "设置寻峰范围"("Enable"=TRUE) -> ("偏移量"=w228:string, "峰7"=w229:string, "峰6"=w230:string, "峰5"=w231:string, "峰4"=w232:string, "峰3"=w233:string, "峰2"=w234:string, "峰1"=w235:string, "确定"=w237:bool)  [unwired: 9 in, 1 out]
                        n96 = Format Into String(format string="峰1：%s\n峰2：%s\n峰3：%s\n峰4：%s\n峰5：%s\n峰6：%s\n峰7：%s\n偏移量：%s" ("格式字符串"), initial string=w223, w235, w234, w233, w232, w231, w230, w229, w228) -> (resulting string=w222:refnum<file>)  [unwired: 1 in, 1 out]
                        n97 = case shown="真" w237 {
                          tunnel: w222 -> [_ w257]
                          tunnel: [TRUE w239] -> w226
                          frame False {
                          }
                          frame True {
                            n98 = Scan From String("峰1：%d-%d\n峰2：%d-%d\n峰3：%d-%d\n峰4：%d-%d\n峰5：%d-%d\n峰6：%d-%d\n峰7：%d-%d\n偏移量：%d" ("格式字符串"), w257) -> (w256:errorcluster, output 1=w242:i32, output 2=w243:i32, output 3=w244:i32, output 4=w245:i32, output 5=w246:i32, output 6=w247:i32, output 7=w248:i32, output 8=w249:i32, output 9=w250:i32, output 10=w251:i32, output 11=w252:i32, output 12=w253:i32, output 13=w254:i32, output 14=w255:i32, output 15=w241:i32)  [unwired: 16 in, 1 out]
                            n99 = case shown="无错误" w256 {
                              tunnel: w241 -> [w278 _]
                              tunnel: w242 -> [w277 _]
                              tunnel: w243 -> [w276 _]
                              tunnel: w244 -> [w275 _]
                              tunnel: w245 -> [w274 _]
                              tunnel: w246 -> [w273 _]
                              tunnel: w247 -> [w272 _]
                              tunnel: w248 -> [w271 _]
                              tunnel: w249 -> [w270 _]
                              tunnel: w250 -> [w269 _]
                              tunnel: w251 -> [w268 _]
                              tunnel: w252 -> [w267 _]
                              tunnel: w253 -> [w266 _]
                              tunnel: w254 -> [w265 _]
                              tunnel: w255 -> [w264 _]
                              tunnel: [TRUE FALSE] -> w239
                              frame No Error {
                                n100 = local write "偏移量"(w278) -> ()
                                n101 = Bundle(w277, w276, w275, w274, w273, w272, w271, w270, w269, w268, w267, w266, w265, w264) -> (w263:T16)  [unwired: 1 in]
                                n102 = Cluster To Array(cluster=w263) -> (array=w262:i32[])
                                n103 = Reshape Array(w262, 7 ("维数大小"), 2 ("维数大小")) -> (w259:i32[][])
                                n104 = local write "峰值范围"(w259) -> ()
                              }
                              frame Error {
                                n105 = One Button Dialog(message="输入格式不符合要求！" ("消息")) -> ()  [unwired: 1 in, 1 out]
                              }
                            }
                          }
                        }
                      }
                    }
                    frame "查看当前设置" {
                      n106 = local read "配置文件路径"() -> (w282:path)
                      n107 = Read from Text File(file (use dialog)=w282) -> (text=w283:string)  [unwired: 3 in, 3 out]
                      n108 = One Button Dialog "单按钮对话框"(message=w283) -> ()  [unwired: 1 in, 1 out]
                    }
                  }
                }
                event "自动寻峰": Value Change {
                  n109 = event-data() -> ()  [unwired: 1 in, 4 out]
                  n110 = local read "峰值Pixel"() -> (w388:dbl[])
                  n111 = local read "峰值波长"() -> (w389:dbl[])
                  n112 = local read "峰值范围"() -> (w344:i32[][])
                  n113 = call <vilib>:"Correlation Coefficient.vi"("Y"=w389, "X"=w388) -> ("r^2"=w387:dbl)  [unwired: 8 in, 1 out]
                  n114 = Index Array(array=w344, index (row)=1 ("索引 (行)")) -> (element=w346:i32[])  [unwired: 1 in]
                  n115 = Index Array(array=w344, index (row)=0 ("索引 (行)")) -> (element=w378:i32[])  [unwired: 1 in]
                  n116 = local write "r^2"(w387) -> ()
                  n117 = Subtract(x=w346, y=w378) -> (x-y=w354:i32[])
                  n118 = Index Array(array=w378, index=0 ("索引")) -> (element=w379:i32)
                  n119 = Index Array(array=w378, index=1 ("索引")) -> (element=w380:i32)
                  n120 = Index Array(array=w378, index=2 ("索引")) -> (element=w381:i32)
                  n121 = Index Array(array=w378, index=3 ("索引")) -> (element=w382:i32)
                  n122 = Index Array(array=w378, index=4 ("索引")) -> (element=w383:i32)
                  n123 = Index Array(array=w378, index=5 ("索引")) -> (element=w384:i32)
                  n124 = Index Array(array=w378, index=6 ("索引")) -> (element=w385:i32)
                  n125 = Index Array(array=w354, index=0 ("索引")) -> (element=w364:i32)
                  n126 = Index Array(array=w354, index=1 ("索引")) -> (element=w365:i32)
                  n127 = Index Array(array=w354, index=2 ("索引")) -> (element=w366:i32)
                  n128 = Index Array(array=w354, index=3 ("索引")) -> (element=w367:i32)
                  n129 = Index Array(array=w354, index=4 ("索引")) -> (element=w368:i32)
                  n130 = Index Array(array=w354, index=5 ("索引")) -> (element=w369:i32)
                  n131 = Index Array(array=w354, index=6 ("索引")) -> (element=w370:i32)
                  n132 = Array Subset(array=w286, index=w379, length=w364) -> (w333:i64[])
                  n133 = Array Subset(array=w286, index=w380, length=w365) -> (w334:i64[])
                  n134 = Array Subset(array=w286, index=w381, length=w366) -> (w335:i64[])
                  n135 = Array Subset(array=w286, index=w382, length=w367) -> (w336:i64[])
                  n136 = Array Subset(array=w286, index=w383, length=w368) -> (w337:i64[])
                  n137 = Array Subset(array=w286, index=w384, length=w369) -> (w338:i64[])
                  n138 = Array Subset(array=w286, index=w385, length=w370) -> (w339:i64[])
                  n139 = Sort 1D Array(array=w333) -> (sorted array=w287:i64[])
                  n140 = Sort 1D Array(array=w334) -> (sorted array=w291:i64[])
                  n141 = Sort 1D Array(array=w335) -> (sorted array=w294:i64[])
                  n142 = Sort 1D Array(array=w336) -> (sorted array=w297:i64[])
                  n143 = Sort 1D Array(array=w337) -> (sorted array=w302:i64[])
                  n144 = Sort 1D Array(array=w338) -> (sorted array=w305:i64[])
                  n145 = Sort 1D Array(array=w339) -> (sorted array=w310:i64[])
                  n146 = Reverse 1D Array(array=w287) -> (reversed array=w317:i64[])
                  n147 = Reverse 1D Array(array=w291) -> (reversed array=w322:i64[])
                  n148 = Reverse 1D Array(array=w294) -> (reversed array=w324:i64[])
                  n149 = Reverse 1D Array(array=w297) -> (reversed array=w326:i64[])
                  n150 = Reverse 1D Array(array=w302) -> (reversed array=w328:i64[])
                  n151 = Reverse 1D Array(array=w305) -> (reversed array=w330:i64[])
                  n152 = Reverse 1D Array(array=w310) -> (reversed array=w332:i64[])
                  n153 = Index Array(array=w317, index=0 ("索引")) -> (element=w316:i64)
                  n154 = Index Array(array=w322, index=0 ("索引")) -> (element=w321:i64)
                  n155 = Index Array(array=w324, index=0 ("索引")) -> (element=w323:i64)
                  n156 = Index Array(array=w326, index=0 ("索引")) -> (element=w325:i64)
                  n157 = Index Array(array=w328, index=0 ("索引")) -> (element=w327:i64)
                  n158 = Index Array(array=w330, index=0 ("索引")) -> (element=w329:i64)
                  n159 = Index Array(array=w332, index=0 ("索引")) -> (element=w331:i64)
                  n160 = Search 1D Array(1D array=w333, element=w316) -> (index of element=w355:i32)  [unwired: 1 in]
                  n161 = Search 1D Array(1D array=w334, element=w321) -> (index of element=w356:i32)  [unwired: 1 in]
                  n162 = Search 1D Array(1D array=w335, element=w323) -> (index of element=w357:i32)  [unwired: 1 in]
                  n163 = Search 1D Array(1D array=w336, element=w325) -> (index of element=w358:i32)  [unwired: 1 in]
                  n164 = Search 1D Array(1D array=w337, element=w327) -> (index of element=w359:i32)  [unwired: 1 in]
                  n165 = Search 1D Array(1D array=w338, element=w329) -> (index of element=w360:i32)  [unwired: 1 in]
                  n166 = Search 1D Array(1D array=w339, element=w331) -> (index of element=w361:i32)  [unwired: 1 in]
                  n167 = Initialize Array(0.0 ("元素"), 7 ("维数大小")) -> (w319:dbl[])
                  n168 = Insert Into Array(array=w319, index=0 ("索引"), new element=w355) -> (w318:dbl[])
                  n169 = Insert Into Array(array=w318, index=1 ("索引"), new element=w356) -> (w300:dbl[])
                  n170 = Insert Into Array(array=w300, index=2 ("索引"), new element=w357) -> (w301:dbl[])
                  n171 = Insert Into Array(array=w301, index=3 ("索引"), new element=w358) -> (w308:dbl[])
                  n172 = Insert Into Array(array=w308, index=4 ("索引"), new element=w359) -> (w309:dbl[])
                  n173 = Insert Into Array(array=w309, index=5 ("索引"), new element=w360) -> (w313:dbl[])
                  n174 = Insert Into Array(array=w313, index=6 ("索引"), new element=w361) -> (w362:dbl[])
                  n175 = local read "偏移量"() -> (w386:i32)
                  n176 = Add(x=w362, y=w378) -> (x+y=w363:dbl[])
                  n177 = Delete From Array(array=w363, length=7 ("长度"), index=7 ("索引")) -> (array with subset deleted=w340:dbl[])  [unwired: 1 out]
                  n178 = Initialize Array(w386, 7 ("维数大小")) -> (w342:i32[])
                  n179 = Add(x=w340, y=w342) -> (x+y=w285:dbl[])
                  n180 = local write "峰值Pixel"(w285) -> ()
                }
              }
              n181 = Build Cluster Array(w189, w182) -> (w199:cluster{dbl, i64}[])
              n182 = Bundle(950, 540) -> (w205:cluster{i32, i32})  [unwired: 1 in]
              n183 = Insert Into Array(array=w187, index=0 ("索引"), new element=w189) -> (w195:dbl[])
              n184 = call <vilib>:"Plot XY.vi"("picture"=w184, "data"=w199, "dimensions (w,h)"=w205, "top left point(0, 0)"=cluster{"x":i16, "y":i16} {"x"=36, "y"=9}, "cartesian axis attributes"="cartesian axis attributes", "cartesian grid cosmetics"=T12 {"line color"=15198183, "text color"=0, "tick length(3)"=3, "crossing axes"=FALSE, "visible grid?"=TRUE}, "XY plot cosmetics"=T11 {"plot color"=16719378, "XY plot type"=enum."connected points", "baseline"=0.0}) -> ("new picture"=→"波形XY图":picture)  [unwired: 8 in]
              n185 = Reshape Array(w195, 2 ("维数大小"), 3649 ("维数大小")) -> (w192:dbl[][])
              n186 = call "转换至动态数据"("2D Array"=w192) -> ("Dynamic Data Type"=w197:dynamicdata)  [unwired: 3 in]
              n187 = call "写入测量文件"("Signals"=w197, "Enable"="导出文本", "Filename"="数据存储路径") -> ()  [unwired: 14 in, 3 out]
              n188 = Or(x="Stop", y="确定") -> (x .or. y?=w177:bool)
              n189 = And(x="确定", y=w179) -> (x .and. y?=w180:bool)
              n190 = Not(x=w179) -> (.not. x?=w178:bool)
              n191 = Or(x=w178, y=w177) -> (x .or. y?=w176:bool)
              n192 = node-c288() -> ()  [unwired: 1 in, 1 out]
            }
            n193 = local write "峰值波长"(dbl[] [631.9517664, 630.1200213, 628.1804588, 576.6350095, 564.9719914, 563.8888147, 558.2540165] ("Y")) -> ()
            n194 = call <vilib>:"Draw Text at Point.vi"("text orientation"=T9."Counterclockwise", "[user-specified font]"=T7 {"Font Name:"="Arial Black", "Size"=22, "Strikeout?"=FALSE, "Italic?"=FALSE, "Underline?"=FALSE, "Outline?"=FALSE, "Shadow?"=FALSE, "Bold?"=TRUE}, "desired font(Application)"=T8."User-specified Font", "text"="Intensity", "origin"=cluster{"x":i16, "y":i16} {"x"=3, "y"=220}) -> ("new picture"=w150:picture)  [unwired: 5 in, 1 out]
            n195 = call <vilib>:"Draw Text at Point.vi"("text orientation"=T9."None", "[user-specified font]"=T7 {"Font Name:"="Arial Black", "Size"=22, "Strikeout?"=FALSE, "Italic?"=FALSE, "Underline?"=FALSE, "Outline?"=FALSE, "Shadow?"=FALSE, "Bold?"=TRUE}, "desired font(Application)"=T8."User-specified Font", "text"="Pixel", "origin"=cluster{"x":i16, "y":i16} {"x"=490, "y"=550}, "picture"=w150) -> ("new picture"=→"pixel picture":picture)  [unwired: 4 in, 1 out]
            n196 = call <vilib>:"Draw Text at Point.vi"("text orientation"=T9."None", "[user-specified font]"=T7 {"Font Name:"="Arial Black", "Size"=22, "Strikeout?"=FALSE, "Italic?"=FALSE, "Underline?"=FALSE, "Outline?"=FALSE, "Shadow?"=FALSE, "Bold?"=TRUE}, "desired font(Application)"=T8."User-specified Font", "text"="Raman Shift(cm-1)", "origin"=cluster{"x":i16, "y":i16} {"x"=430, "y"=550}, "picture"=w150) -> ("new picture"=→"λ picture":picture)  [unwired: 4 in, 1 out]
            n197 = node-c288(w169) -> ()  [unwired: 1 out]
            n198 = case shown="假" w168 {
              tunnel: [w174 w175] -> w171
              frame False {
                w174 = 状态机."Init"  # 枚举
              }
              frame True {
                w175 = 状态机."GetData"  # 枚举
              }
            }
          }
        }
      }
      frame "Exit" {
        w422 = 状态机."Init"  # 枚举
        n199 = local read "采集状态"() -> (w420:bool)
        n200 = case shown="假" w420 {
          frame False {
          }
          frame True {
            n201 = local write "采集状态"(FALSE ("打开状态")) -> ()
            n202 = local read "串口名"() -> (w423:T4)
            n203 = VISA Close(VISA resource name=w423) -> ()  [unwired: 1 in, 1 out]
          }
        }
      }
    }
    "Debug状态" <- w5
    n204 = Or(x=w4, y="关闭串口并退出") -> (x .or. y?=w2:bool)
  }
